vi "Fit Cubic Spline + Sine.vi"(0 "Decay":cluster{"t Axis":dbl[], "Y axis":dbl[]}, 1 "Optimal Offset Selection Criterion":T1, 7 "Cubic Spline + Sine Options":T2, 9 "Basic Fit Options":T3, 11 "error in (no error)":errorcluster) -> (4 "Fitted Decay":cluster{"t Array":dbl[], "Fitted Array":dbl[]}, 6 "Residuals":cluster{"t Array":dbl[], "Residual Array":dbl[]}, 8 "Fit Output":T8={"best nonlinear fit"=[], "best fit parameters"=[], "R^2"=0.0, "RMSE"=0.0, "error out"={"status"=FALSE, "code"=0, "source"=""}, "Fitting Method"=enum."Least Square", "number of function calls"=0, "number of iterations"=0, "covariance"=[], "Chi 2"=0.0, "DOF"=0, "Fit Convergence Criterion"=enum."Continue", "Fitting Algorithm"=enum."Levenberg-Marquardt", "Weighted Fit"=enum."Unweighted", "Gradient"=0.0, "|Delta Chi 2|"=0.0, "|Delta Chi 2|/Chi 2"=0.0, "Max |Delta a| /|a|"=0.0, "Lambda"=-1.0, "RSS"=0.0, "AIC"=0.0, "BIC"=0.0, "Max number of function calls"=0, "Max number of iterations"=0, "IRF"={"X Array"=[], "Y Array"=[]}, "IRF Normalization Factor"=0.0, "Decay Normalization Factor"=0.0, "Number of offset fits"=0, "Weighted Chi2"=-1.0, "Unweighted Chi2"=-1.0}, 10 "Delta Best Fit Parameters":dbl[](array[numeric]), 15 "error out":errorcluster)   [LabVIEW 2021, in "Fits.lvlib"]
uses:
  Fits.lvlib
  Non-linear Fit Output v4.ctl
  Nonlinear Fit Method.ctl
  <vilib>/Analysis/Matrix/Datatypes/RealMatrix.ctl
  Convergence Criteria.ctl
  Non-linear Fitting Algorithm.ctl
  IRF(X)PSED/Fit Weights Type v2.ctl
  Graphs/XY Graph/XY Graph Plot Data.ctl
  Basic Fit Options.ctl
  Non-linear Fitting Method v2.ctl
  Residual Type.ctl
  Cubic Spline + Sine Options.ctl
  Optimal Offset Selection Criterion.ctl
  LM Cubic Spline + Sine and gradient.vi
  <vilib>/Utility/error.llb/Error Cluster From Error Code.vi
  <vilib>/ErrorRing/Error Ring.xnode
  Time/Time.lvlib
  <vilib>/Analysis/Matrix/NI_Matrix.lvlib
  Graphs/XY Graph/XY Graph Add-Ons.lvlib
panel:
  out "XY Graph":cluster{"X Array":dbl[], "Y Array":dbl[]}[](graph)
  out "CPU (s)":dbl
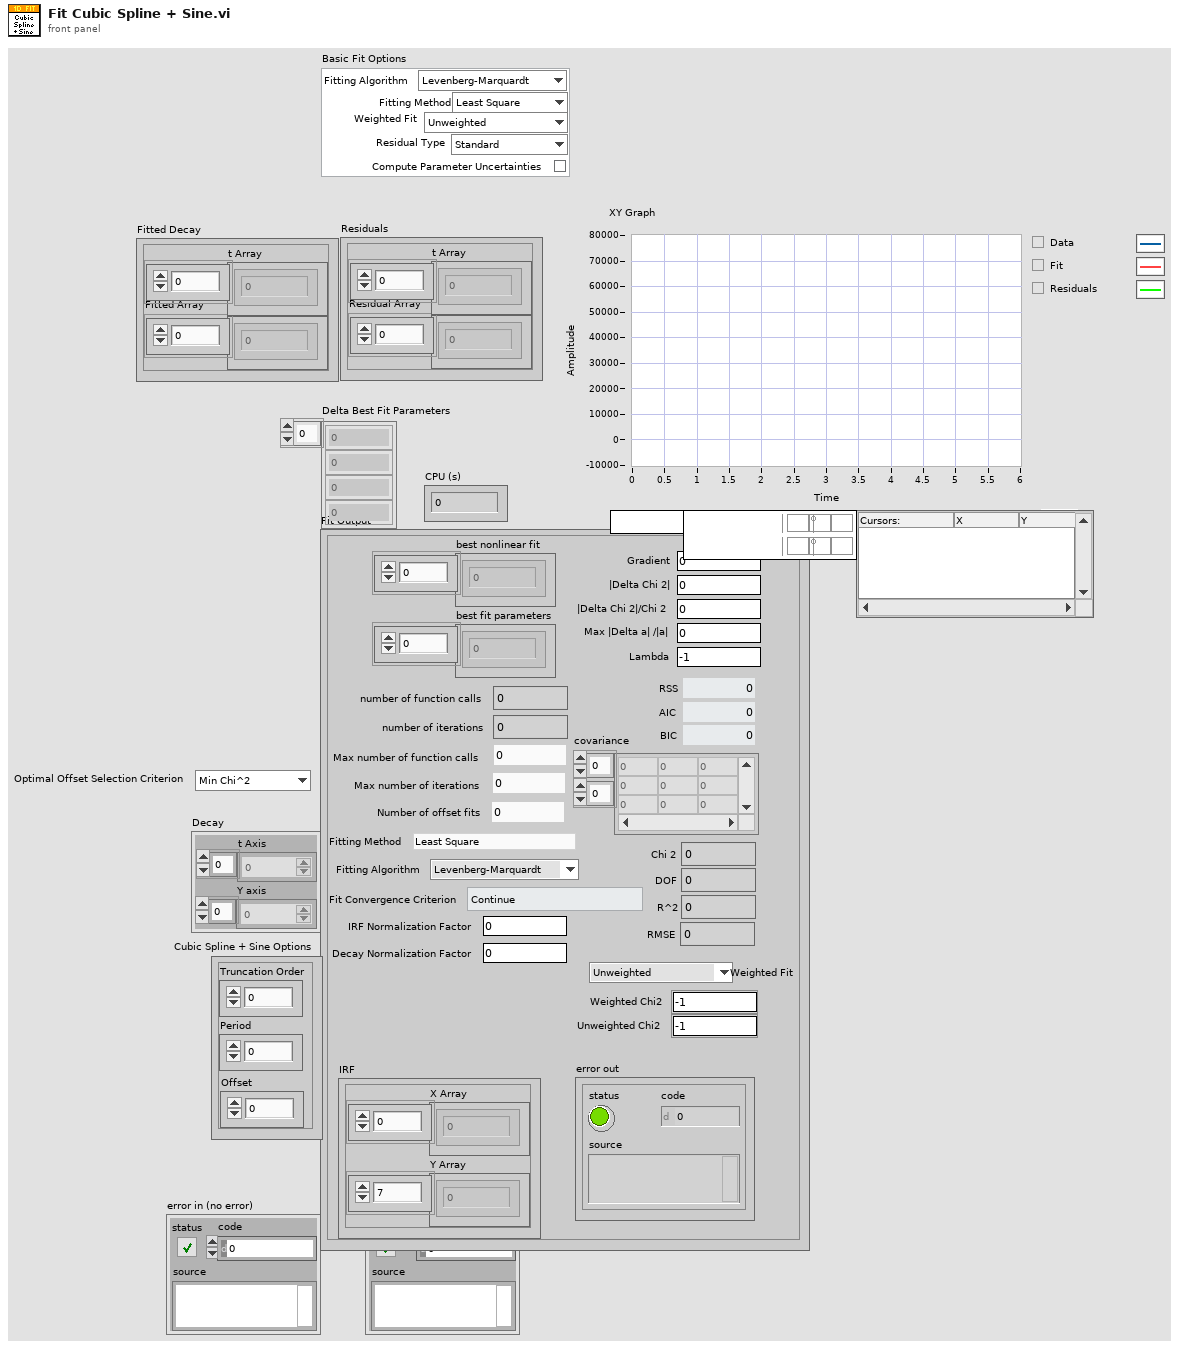
[diagram p1: front panel]
types:
  T1 = typedef "Fits.lvlib/Optimal Offset Selection Criterion.ctl" = enum16{"Min Chi^2", "Max R^2"}
  T2 = typedef "Fits.lvlib/Cubic Spline + Sine Options.ctl" = cluster{"Truncation Order":i32, "Period":dbl, "Offset":dbl}
  T3 = typedef "Fits.lvlib/Basic Fit Options.ctl" = cluster{"Fitting Method":T4, "Weighted Fit":T5, "Residual Type":T6, "Compute Parameter Uncertainties":bool, "Fitting Algorithm":T7}
  T4 = typedef "Fits.lvlib/Non-linear Fitting Method v2.ctl" = enum16{"Least Square", "Least Absolute Residual", "Bisquare", "MLE", "-", "Best of All"}
  T5 = typedef "Fits.lvlib/Fit Weights Type v2.ctl" = enum16{"Unweighted", "1/Variance (Neyman)", "1/Variance (Pearson)", "Best of All"}
  T6 = typedef "Fits.lvlib/Residual Type.ctl" = enum16{"Standard", "Normalized", "Reduced"}
  T7 = typedef "Fits.lvlib/Non-linear Fitting Algorithm.ctl" = enum16{"Levenberg-Marquardt", "Trust-Region Dogleg"}
  T8 = typedef "Fits.lvlib/Non-linear Fit Output v4.ctl" = cluster{"best nonlinear fit":dbl[], "best fit parameters":dbl[], "R^2":dbl, "RMSE":dbl, "error out":errorcluster, "Fitting Method":T9, "number of function calls":i32, "number of iterations":i32, "covariance":T10, "Chi 2":dbl, "DOF":i32, "Fit Convergence Criterion":T11, "Fitting Algorithm":T7, "Weighted Fit":T5, "Gradient":dbl, "|Delta Chi 2|":dbl, "|Delta Chi 2|/Chi 2":dbl, "Max |Delta a| /|a|":dbl, "Lambda":dbl, "RSS":dbl, "AIC":dbl, "BIC":dbl, "Max number of function calls":i32, "Max number of iterations":i32, "IRF":T12, "IRF Normalization Factor":dbl, "Decay Normalization Factor":dbl, "Number of offset fits":i32, "Weighted Chi2":dbl, "Unweighted Chi2":dbl}
  T9 = typedef "Fits.lvlib/Nonlinear Fit Method.ctl" = enum16{"Least Square", "Least Absolute Residual", "Bisquare", "MLE"}
  T10 = typedef "NI_Matrix.lvlib/RealMatrix.ctl" = dbl[][]
  T11 = typedef "Fits.lvlib/Convergence Criteria.ctl" = enum16{"Continue", "Tolerances Exceeded", "Max Time Exceeded", "Max Iterations Exceeded", "Max Function Evaluations Exceeded", "Scale Range Exceeded"}
  T12 = typedef "XY Graph Add-Ons.lvlib/XY Graph Plot Data.ctl" = cluster{"X Array":dbl[], "Y Array":dbl[]}
  T13 = cluster{"parameter minimum":dbl[], "parameter maximum":dbl[]}
  T14 = cluster{"t Axis":dbl[], "best nonlinear fit":dbl[]}
  T15 = cluster{"t Axis":dbl[], "best nonlinear fit":dbl[]}[]
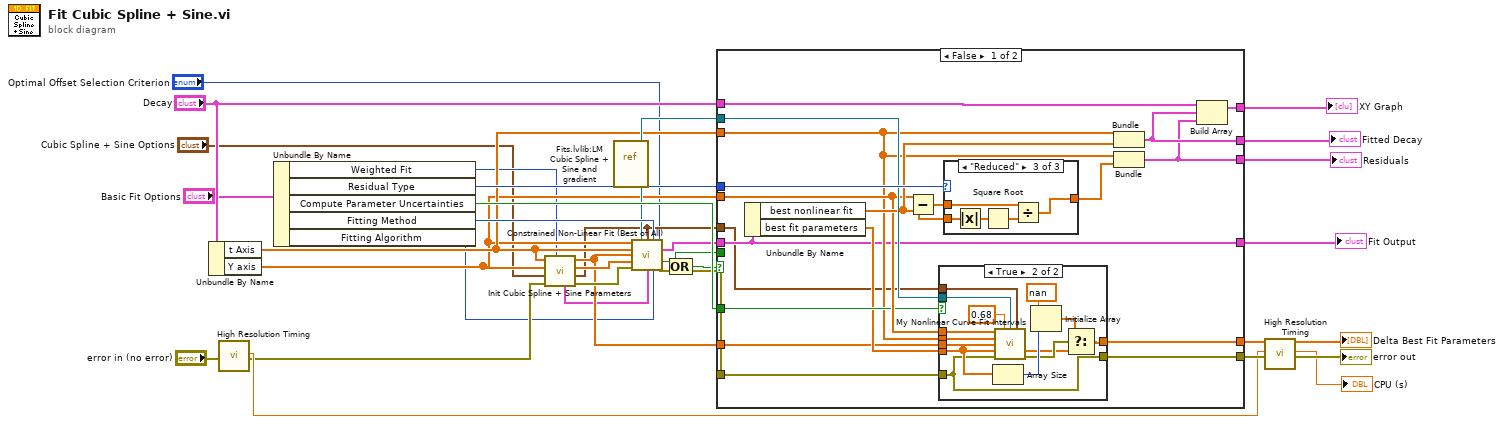
[diagram p0: block diagram]
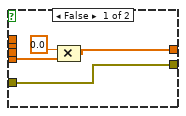
[diagram p2: hidden frame]
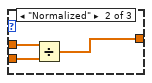
[diagram p4: hidden frame]
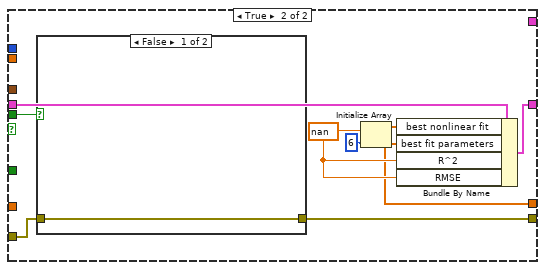
[diagram p5: hidden frame]
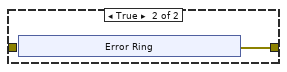
[diagram p6: hidden frame]
diagram:
  n1 = Unbundle By Name("Decay") -> ("t Axis"=w13:dbl[], "Y axis"=w12:dbl[])
  n2 = call "High Resolution Timing.vi"("Error In"="error in (no error)") -> ("elapsed (relative) seconds"=w15:dbl, "Error Out"=w11:errorcluster)  [unwired: 16 in, 1 out]
  n3 = Unbundle By Name("Basic Fit Options") -> ("Weighted Fit"=w9:T5, "Residual Type"=w29:T6, "Compute Parameter Uncertainties"=w30:bool, "Fitting Method"=w32:T4, "Fitting Algorithm"=w3:T7)
  n4 = call "Init Cubic Spline + Sine Parameters.vi"("Weighted Fit"=w9, "error in (no error)"=w11, "Cubic Spline + Sine Options"="Cubic Spline + Sine Options", "Y axis in"=w12, "t Axis in"=w13) -> ("error out"=w10:errorcluster, "Cubic Spline + Sine Options"=w4:T2, "Initial Parameters"=w8:dbl[], "Weights"=w7:dbl[], "parameter bounds"=w6:T13)  [unwired: 2 in]
  n5 = vi-ref "Fits.lvlib:LM Cubic Spline + Sine and gradient.vi"() -> (w14:refnum<vi>)
  n6 = call "Constrained Non-Linear Fit (Best of All).vi"("Y Array"=w12, "f(x,a)"=w14, "Data"=w4, "Fitting Method"=w32, "Optimal Offset Selection Criterion"="Optimal Offset Selection Criterion", "X Array"=w13, "Weights"=w7, "Guess Fitted Parameters"=w8, "error in (no error)"=w10, "Fitted parameter bounds"=w6, "Fitting Algorithm"=w3) -> ("Fit Output"=w2:T8, "Fit Aborted?"=w17:bool, "Error Out"=w18:errorcluster)  [unwired: 1 in, 1 out]
  n7 = Compound Arithmetic op=OR(w17, w18) -> (w19:bool)
  n8 = case shown="False" w19 {
    tunnel: "Decay" -> [w51 _]
    tunnel: [w50 _] -> w22
    tunnel: [w49 _] -> w26
    tunnel: [w48 w84] -> w16
    tunnel: [w47 w80] -> w25
    tunnel: [w46 _] -> w27
    tunnel: w29 -> [w45 _]
    tunnel: w13 -> [w38 _]
    tunnel: w14 -> [w42 _]
    tunnel: w12 -> [w40 _]
    tunnel: w2 -> [w35 w83]
    tunnel: w18 -> [w36 w85]
    tunnel: [w35 w82] -> w28
    tunnel: w30 -> [w39 _]
    tunnel: w17 -> [_ w79]
    tunnel: w4 -> [w34 _]
    tunnel: w7 -> [w33 _]
    frame False {
      n9 = Unbundle By Name(w35) -> ("best nonlinear fit"=w41:dbl[], "best fit parameters"=w37:dbl[])
      n10 = Subtract(x=w40, y=w41) -> (x-y=w44:dbl[])
      n11 = case shown="True" w39 {
        tunnel: [w55 w58] -> w48
        tunnel: [w53 w59] -> w47
        tunnel: w38 -> [_ w68]
        tunnel: w42 -> [_ w67]
        tunnel: w37 -> [w54 w65]
        tunnel: w40 -> [_ w66]
        tunnel: w36 -> [w55 w58]
        tunnel: w34 -> [_ w57]
        tunnel: w33 -> [_ w56]
        frame False {
          n12 = Compound Arithmetic op=MULTIPLY(0.0, w54) -> (w53:dbl[])
        }
        frame True {
          n13 = Array Size(array=w65) -> (size(s)=w64:i32)
          n14 = call "My Nonlinear Curve Fit Intervals.vi"("Y"=w66, "confidence level"=0.68, "f(x,a)"=w67, "data"=w57, "X"=w68, "Weight"=w56, "best fit parameters"=w65, "error in (no error)"=w58) -> ("delta best fit parameters"=w60:dbl[], "error out"=w61:errorcluster)  [unwired: 6 in]
          n15 = Initialize Array(nan ("element"), w64) -> (w62:dbl[])
          n16 = Select(t=w62, s=w61, f=w60) -> (s? t:f=w59:dbl[])
        }
      }
      n17 = case shown="\"Reduced\"" w45 {
        tunnel: w44 -> [w70 w73 w78]
        tunnel: [w70 w71 w76] -> w43
        tunnel: w41 -> [_ w72 w77]
        frame "Standard", Default {
        }
        frame "Normalized" {
          n18 = Divide(x=w73, y=w72) -> (x/y=w71:dbl[])
        }
        frame "Reduced" {
          n19 = Absolute Value(x=w77) -> (abs(x)=w75:dbl[])
          n20 = Square Root(x=w75) -> (sqrt(x)=w74:dbl[])
          n21 = Divide(x=w78, y=w74) -> (x/y=w76:dbl[])
        }
      }
      n22 = Bundle("t Axis"=w38, "best nonlinear fit"=w41) -> (w49:T14)  [unwired: 1 in]
      n23 = Bundle("t Axis"=w38, w43) -> (w46:cluster{"t Axis":dbl[], dbl[]})  [unwired: 1 in]
      n24 = Build Array(w51, w49, w46) -> (w50:T15)
    }
    frame True {
      w81 = nan ("element")
      n25 = case shown="False" w79 {
        tunnel: w85 -> [w87 _]
        tunnel: [w87 w88] -> w84
        frame False {
        }
        frame True {
          n26 = xnode "Error Ring"() -> ("error out"=w88:errorcluster)
        }
      }
      n27 = Initialize Array(w81, 6 ("dimension size")) -> (w80:dbl[])
      n28 = Bundle By Name(cluster=w83, "best nonlinear fit"=w80, "best fit parameters"=w80, "R^2"=w81, "RMSE"=w81) -> (w82:T8)
    }
  }
  "Fit Output" <- w28
  "Residuals" <- w27
  "Fitted Decay" <- w26
  "Delta Best Fit Parameters" <- w25
  "XY Graph" <- w22
  n29 = call "High Resolution Timing.vi"("relative seconds (NaN)"=w15, "Error In"=w16) -> ("elapsed (relative) seconds"=→"CPU (s)":dbl, "Error Out"=→"error out":errorcluster)  [unwired: 15 in, 1 out]
